vi "TestPlan - Config File.vi"(6 "Action":enum16{"Write", "Read", "Read All", "Remove"}(ring), 7 "file path":path, 8 "error in (no error)":errorcluster, 9 "Value":string[](array[string]), 10 "Key Name":string[](array[string]), 11 "TestPlan Section":string) -> (0 "error out":errorcluster, 2 "key names":string[](array[string]), 3 "Value Out":T1(array[cluster]))   [LabVIEW 2019]
uses:
  <vilib>/Utility/config.llb/Write Key (String).vi
  <vilib>/Utility/config.llb/Read Key (String).vi
  <vilib>/Utility/config.llb/NI_LVConfig.lvlib
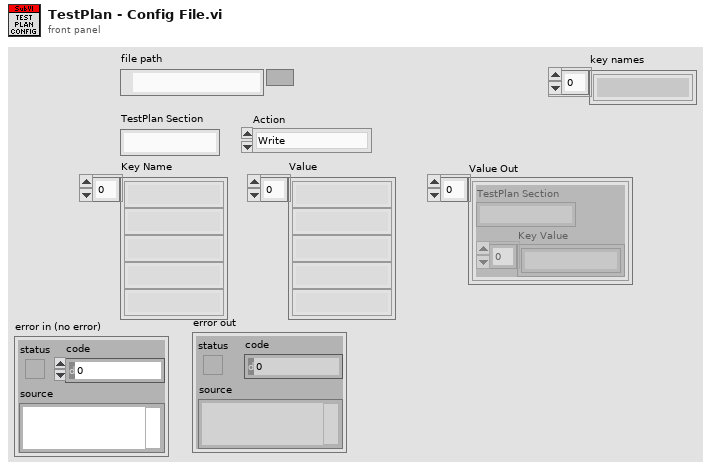
[diagram p1: front panel]
types:
  T1 = cluster{"TestPlan Section":string, "Key Value":string[]}[]
  T2 = typedef "NI_LVConfig.lvlib/Config Data RefNum.ctl" = refnum<k1>
  T3 = cluster{"TestPlan Name":string, "Key Value":string[]}
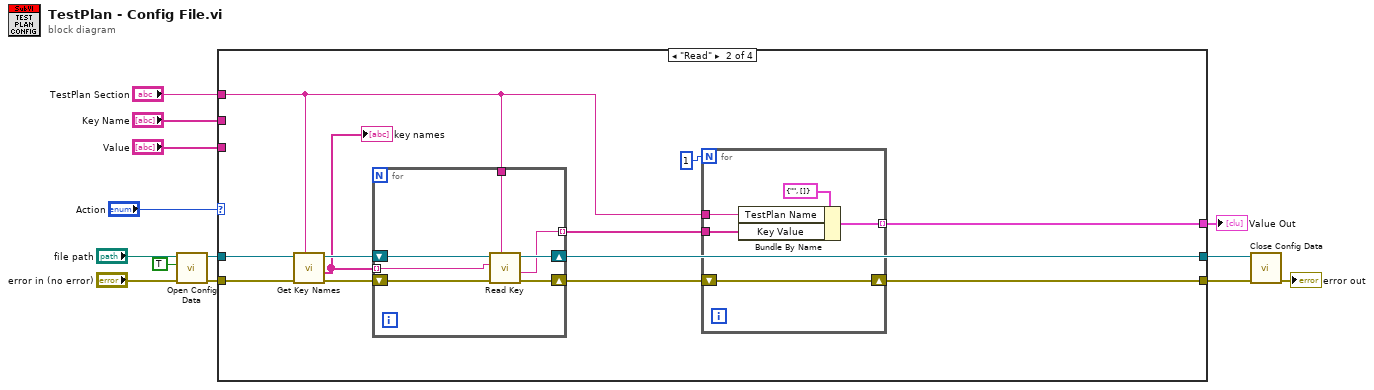
[diagram p0: block diagram]
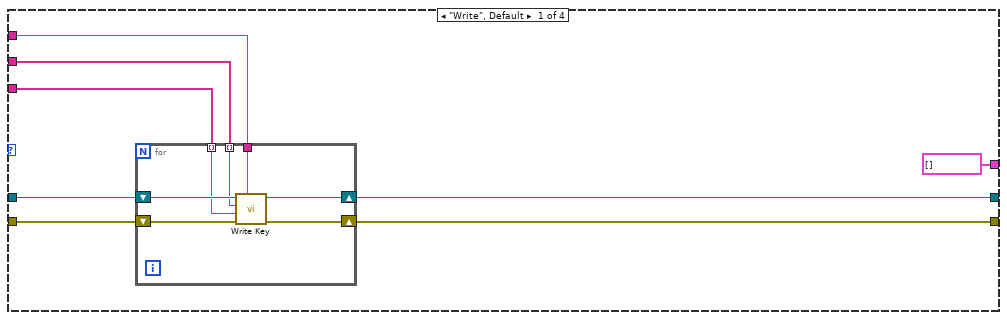
[diagram p2: hidden frame]
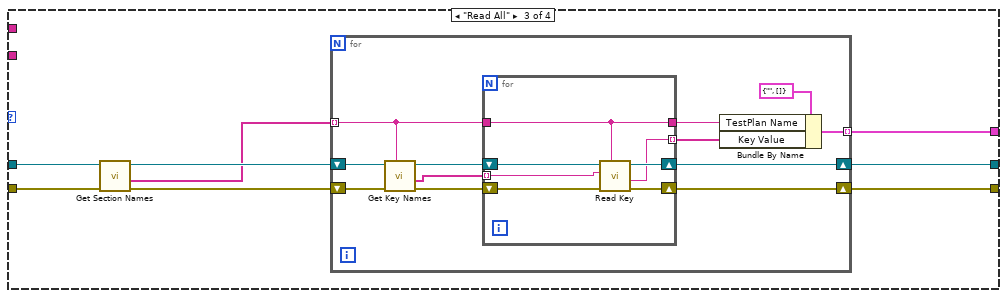
[diagram p3: hidden frame]
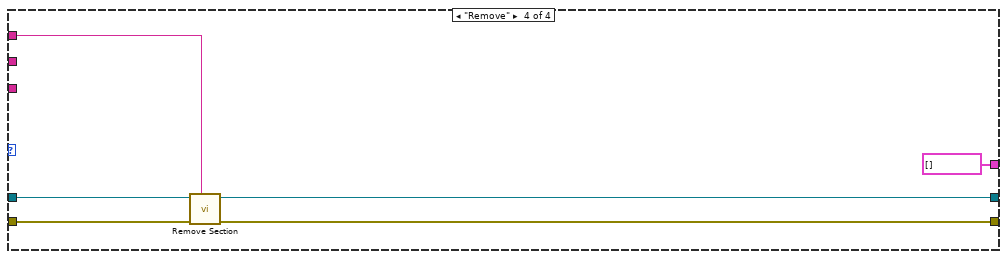
[diagram p4: hidden frame]
diagram:
  n1 = call <vilib>:"Open Config Data.vi"("error in (no error)"="error in (no error)", "create file if necessary (T)"=TRUE, "configuration file path"="file path") -> ("error out"=w13:errorcluster, "refnum"=w12:T2)  [unwired: 6 in, 1 out]
  n2 = case shown="\"Read\"" "Action" {
    tunnel: w13 -> [w21 w33 w57 w83]
    tunnel: w12 -> [w20 w31 w56 w85]
    tunnel: [w19 w40 w59 w84] -> w11
    tunnel: [w18 w36 w60 w82] -> w10
    tunnel: "Value" -> [w17 _ _ _]
    tunnel: "Key Name" -> [w16 _ _ _]
    tunnel: "TestPlan Section" -> [w15 w30 _ w81]
    tunnel: [cluster{"Station Name":string, "Key":string[]}[] [] w38 w58 cluster{"Station Name":string, "Key":string[]}[] []] -> w3
    frame "Write", Default {
      n3 = for {
        shift-right: [w25] -> w18
        shift-left: w21 -> [w28]
        shift-right: [w26] -> w19
        shift-left: w20 -> [w27]
        tunnel: w15 -> [w24]
        tunnel: w16 -> [w23] mode=indexing
        tunnel: w17 -> [w22] mode=indexing
        n4 = call-poly <vilib>:"Write Key.vi"("section"=w24, "error in (no error)"=w28, "value"=w22, "key"=w23, "refnum"=w27) -> ("error out"=w25:errorcluster, "refnum out"=w26:T2)  [unwired: 4 in, 1 out]
      }
    }
    frame "Read" {
      n5 = call <vilib>:"Get Key Names.vi"("section"=w30, "error in (no error)"=w33, "refnum"=w31) -> ("error out"=w34:errorcluster, "key names"=w29:string[], "refnum out"=w32:T2)  [unwired: 5 in, 1 out]
      "key names" <- w29
      n6 = for {
        tunnel: w30 -> [w48]
        shift-right: [w49] -> w40
        shift-left: w32 -> [w52]
        shift-right: [w50] -> w35
        shift-left: w34 -> [w51]
        tunnel: [w47] -> w39 mode=indexing
        tunnel: w29 -> [w46] mode=indexing
        n7 = call-poly <vilib>:"Read Key.vi"("section"=w48, "error in (no error)"=w51, "key"=w46, "refnum"=w52) -> ("error out"=w50:errorcluster, "value"=w47:string, "refnum out"=w49:T2)  [unwired: 4 in, 1 out]
      }
      n8 = for {
        N: 1 -> [_]
        tunnel: w30 -> [w44]
        tunnel: w39 -> [w43]
        tunnel: [w42] -> w38 mode=indexing
        shift-right: [w41] -> w36
        shift-left: w35 -> [w41]
        n9 = Bundle By Name(cluster=T3 {"TestPlan Name"="", "Key Value"=[]}, "TestPlan Name"=w44, "Key Value"=w43) -> (w42:T3)
      }
    }
    frame "Read All" {
      n10 = call <vilib>:"Get Section Names.vi"("error in (no error)"=w57, "refnum"=w56) -> ("error out"=w55:errorcluster, "section names"=w53:string[], "refnum out"=w54:T2)  [unwired: 7 in]
      n11 = for {
        tunnel: [w61] -> w58 mode=indexing
        shift-right: [w72] -> w60
        shift-left: w55 -> [w70]
        shift-right: [w71] -> w59
        shift-left: w54 -> [w68]
        tunnel: w53 -> [w65] mode=indexing
        n12 = call <vilib>:"Get Key Names.vi"("section"=w65, "error in (no error)"=w70, "refnum"=w68) -> ("error out"=w69:errorcluster, "key names"=w66:string[], "refnum out"=w67:T2)  [unwired: 5 in, 1 out]
        n13 = for {
          shift-right: [w76] -> w71
          shift-left: w67 -> [w79]
          shift-right: [w77] -> w72
          shift-left: w69 -> [w78]
          tunnel: [w75] -> w62 mode=indexing
          tunnel: w66 -> [w74] mode=indexing
          tunnel: w65 -> [w73]
          tunnel: [w73] -> w63
          n14 = call-poly <vilib>:"Read Key.vi"("section"=w73, "error in (no error)"=w78, "key"=w74, "refnum"=w79) -> ("error out"=w77:errorcluster, "value"=w75:string, "refnum out"=w76:T2)  [unwired: 4 in, 1 out]
        }
        n15 = Bundle By Name(cluster=T3 {"TestPlan Name"="", "Key Value"=[]}, "TestPlan Name"=w63, "Key Value"=w62) -> (w61:T3)
      }
    }
    frame "Remove" {
      n16 = call <vilib>:"Remove Section.vi"("section"=w81, "error in (no error)"=w83, "refnum"=w85) -> ("error out"=w82:errorcluster, "refnum out"=w84:T2)  [unwired: 6 in, 1 out]
    }
  }
  "Value Out" <- w3
  n17 = call <vilib>:"Close Config Data.vi"("error in (no error)"=w10, "refnum"=w11) -> ("error out"=→"error out":errorcluster)  [unwired: 8 in, 1 out]
